vi "Get Status.vi"(8 "error in":errorcluster) -> (0 "error out":errorcluster, 3 "Messages":i32)   [LabVIEW 2025, in "CAN-LIN Raw Bus Capture UI.lvlib"]
uses:
  CAN-LIN Raw Bus Capture UI.lvlib
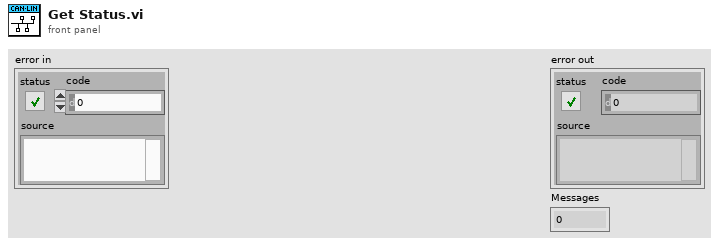
[diagram p1: front panel]
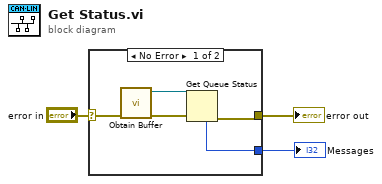
[diagram p0: block diagram]
diagram:
  n1 = case shown="No Error" "error in" {
    selector: "error in" -> [w4 w9]
    tunnel: [w8 w9] -> w2
    tunnel: [w7 _] -> w1
    frame No Error {
      n2 = call "Obtain Buffer.vi"("error in (no error)"=w4) -> ("error out"=w6:errorcluster, "Table Queue"=w5:refnum<queue>)  [unwired: 9 in]
      n3 = Get Queue Status(queue=w5, error in (no error)=w6) -> (error out=w8:errorcluster, # elements in queue=w7:i32)  [unwired: 1 in, 6 out]
    }
    frame Error {
    }
  }
  "error out" <- w2
  "Messages" <- w1
